vi "복합연산2.vi"() -> ()   [LabVIEW 2019]
panel:
  out "D":bool
  in  "C":bool
  in  "B":bool
  in  "A":bool
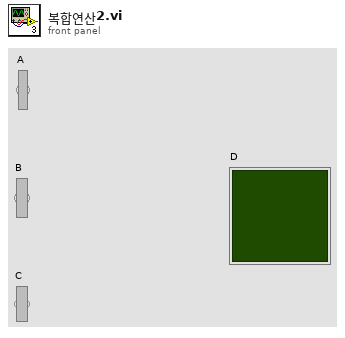
[diagram p1: front panel]
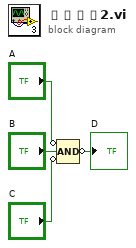
[diagram p0: block diagram]
diagram:
  n1 = Compound Arithmetic op=AND(invert "A", "B", invert "C") -> (invert →"D":bool)
